vi "JAPCtiming2.vi"(8 "error in (no error)":errorcluster) -> (0 "error out":errorcluster)   [LabVIEW 2014]
uses:
  <userlib>/_RADE/RIO/JAPC/classes/JGet/openJAPCGet.vi
  <userlib>/_RADE/RIO/JAPC/classes/JGet/JAPCGet.vi
  <userlib>/_RADE/RIO/JAPC/classes/JGet/JGet.lvclass
panel:
  out "F-format string":string
  out "x-y":u32
  in  "stop":bool
  in  "URL":string
  out "data 2":dbl
  out "Instantaneous data":variant
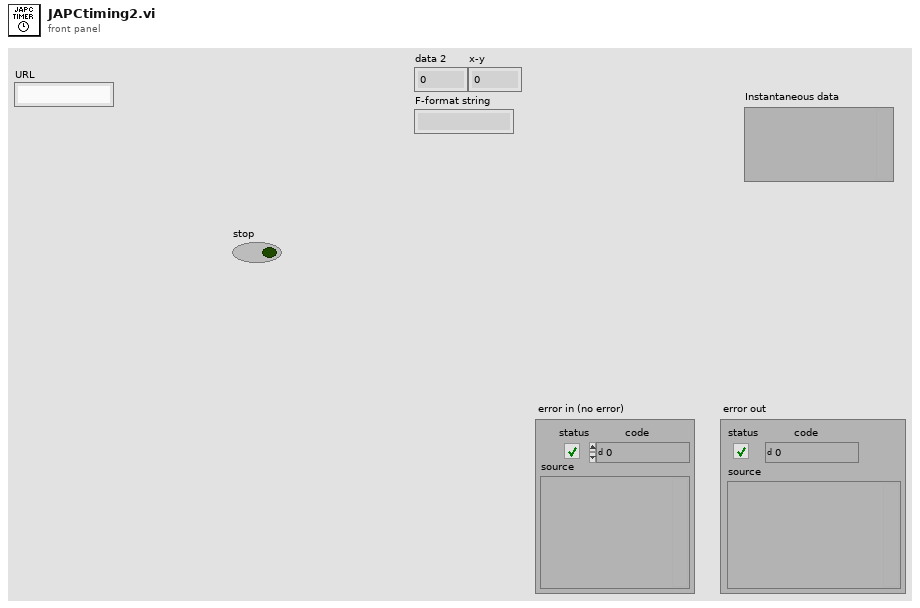
[diagram p1: front panel]
types:
  T1 = enum16{"open", "replace", "create", "open or create", "replace or create", "replace or create with confirmation"}
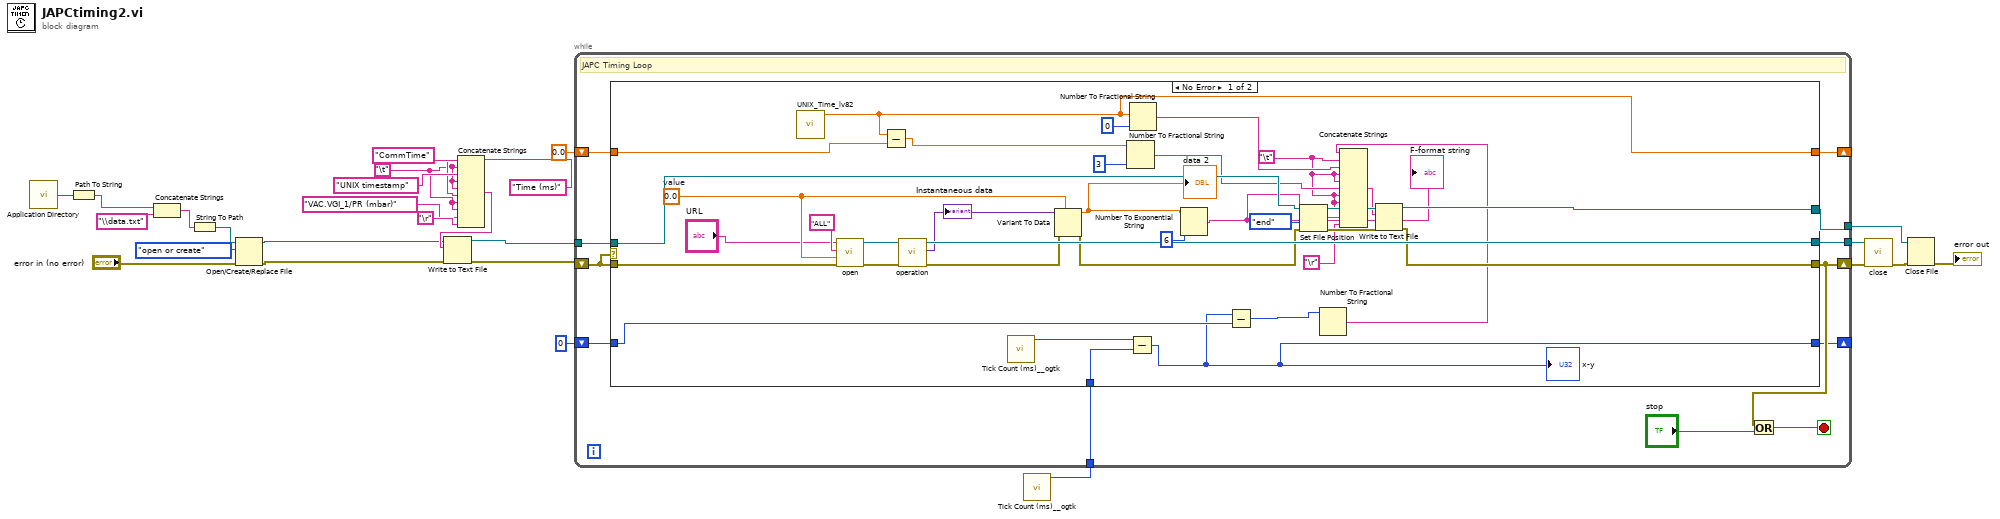
[diagram p0: block diagram]
diagram:
  w2 = "\t"
  n1 = call <vilib>:"Application Directory.vi"() -> ("Application Directory"=w20:path)
  n2 = Path To String(path=w20) -> (string=w19:string)
  n3 = Concatenate Strings(w19, "\\data.txt" ("string")) -> (w16:string)
  n4 = String To Path(string=w16) -> (path=w17:path)
  n5 = Open/Create/Replace File(file path (use dialog)=w17, error in="error in (no error)", operation (0:open)=T1."open or create") -> (refnum out=w7:refnum<file>, error out=w8:errorcluster)  [unwired: 3 in, 1 out]
  n6 = Concatenate Strings("CommTime" ("string"), w2, "UNIX timestamp" ("string"), w2, w2, "Time (ms)" ("string"), w2, w2, "VAC.VGI_1/PR (mbar)" ("string"), "\r") -> (w14:string)
  n7 = Write to Text File(file (use dialog)=w7, text=w14, error in=w8) -> (refnum out=w6:refnum<file>, error out=w9:errorcluster)  [unwired: 1 in, 1 out]
  n8 = call <userlib>:"Tick Count (ms)__ogtk.vi"() -> ("millisecond timer value"=w5:u32)  [unwired: 10 in, 1 out]
  n9 = while {
    tunnel: [w38] -> w26
    shift-right: [w36] -> w25
    shift-left: w9 -> [w35]
    tunnel: [w34] -> w15
    tunnel: w6 -> [w32]
    tunnel: w5 -> [w31]
    shift-right: [w30] -> _
    shift-left: u32 0 -> [w29]
    shift-right: [w28] -> _
    shift-left: 0.0 ("Unix time") -> [w27]
    stop <- w37 stop-if-true
    # "JAPC Timing Loop"
    n10 = case shown="No Error" w35 {
      tunnel: [w73 _] -> w38
      tunnel: [w66 w77] -> w36
      tunnel: w35 -> [w63 w77]
      tunnel: w32 -> [w62 w76]
      tunnel: [w64 w76] -> w34
      tunnel: w31 -> [w54 _]
      tunnel: [w51 w75] -> w30
      tunnel: w29 -> [w52 w75]
      tunnel: [w43 w74] -> w28
      tunnel: w27 -> [w42 w74]
      frame No Error {
        w39 = "\t"
        w72 = 0.0  # value
        n11 = call "UNIX_Time_lv82.vi"() -> ("Unix time"=w43:dbl)  [unwired: 11 in]
        n12 = call-poly <userlib>:"open.vi"("error in (no error)"=w63, "Data type"=w72, "Cycle"="ALL", "URL"="URL") -> ("error out"=w71:errorcluster, "Object out"=w70:refnum<class "JGet.lvclass">)  [unwired: 6 in]
        n13 = Subtract(x=w43, y=w42) -> (x-y=w41:dbl)
        n14 = call-poly <userlib>:"operation.vi"("error in (no error)"=w71, "Object in"=w70) -> ("error out"=w68:errorcluster, "Data"=w67:variant, "Object out"=w73:refnum<class "JGet.lvclass">)  [unwired: 5 in, 2 out]
        "Instantaneous data" <- w67
        n15 = call <userlib>:"Tick Count (ms)__ogtk.vi"() -> ("millisecond timer value"=w53:u32)  [unwired: 10 in, 1 out]
        n16 = Variant To Data(error in=w68, type=w72, Variant=w67) -> (data=w47:dbl, error out=w60:errorcluster)
        "data 2" <- w47
        n17 = Number To Fractional String(number=w41, precision (6)=i16 3) -> (F-format string=w40:string)  [unwired: 2 in]
        n18 = Subtract(x=w53, y=w54) -> (x-y=w51:u32)
        "x-y" <- w51
        n19 = Number To Fractional String(number=w43, precision (6)=i16 0) -> (F-format string=w56:string)  [unwired: 2 in]
        n20 = Number To Exponential String(number=w47, precision (6)=i16 6) -> (E-format string=w48:string)  [unwired: 2 in]
        "F-format string" <- w48
        n21 = Subtract(x=w51, y=w52) -> (x-y=w50:u32)
        n22 = Set File Position(refnum=w62, from (0:start)=enum16{"start", "end", "current"}."end", error in=w60) -> (refnum out=w58:refnum<file>, error out=w59:errorcluster)  [unwired: 1 in]
        n23 = Number To Fractional String(number=w50) -> (F-format string=w49:string)  [unwired: 3 in]
        n24 = Concatenate Strings(w49, w39, w56, w39, w39, w40, w39, w39, w39, w48, "\r") -> (w55:string)
        n25 = Write to Text File(file (use dialog)=w58, text=w55, error in=w59) -> (refnum out=w64:refnum<file>, error out=w66:errorcluster)  [unwired: 1 in, 1 out]
      }
      frame Error {
      }
    }
    n26 = Or(x=w36, y="stop") -> (x .or. y?=w37:bool)
  }
  n27 = call-dynamic "close.vi"("error in (no error)"=w25, "Object in"=w26) -> ("error out"=w24:errorcluster)  [unwired: 9 in]
  n28 = Close File(refnum=w15, error in=w24) -> (error out=→"error out":errorcluster)  [unwired: 1 out]
